vi "graphHandler.vi"(0 "Maxes[wl]":dbl[][](array[numeric]), 4 "Bounds[wl]":dbl[][](array[numeric]), 5 "delta inc":dbl, 6 "deltas":dbl[](array[numeric]), 7 "freq inc":dbl, 8 "wavelengths":dbl[](array[numeric]), 11 "trace (r=wl, c=d)":dbl[][](array[numeric])=array321x127[40767 elements]) -> (1 "Scale mult/offset":T2, 2 "Cursors":T1(array[cluster]), 3 "output trace (r=d, c=freq)":dbl[][](array[numeric]))   [LabVIEW 2022 SP3]
uses:
  <vilib>/gmath/NI_Gmath.lvlib
panel:
  out "resampled deltas":dbl[](array[numeric])
  out "error 2":i32
  out "resampled freqs":dbl[](array[numeric])
  out "Array":dbl[](array[numeric])
  out "error":i32
  out "freqs (rad*PHz)":dbl[](array[numeric])
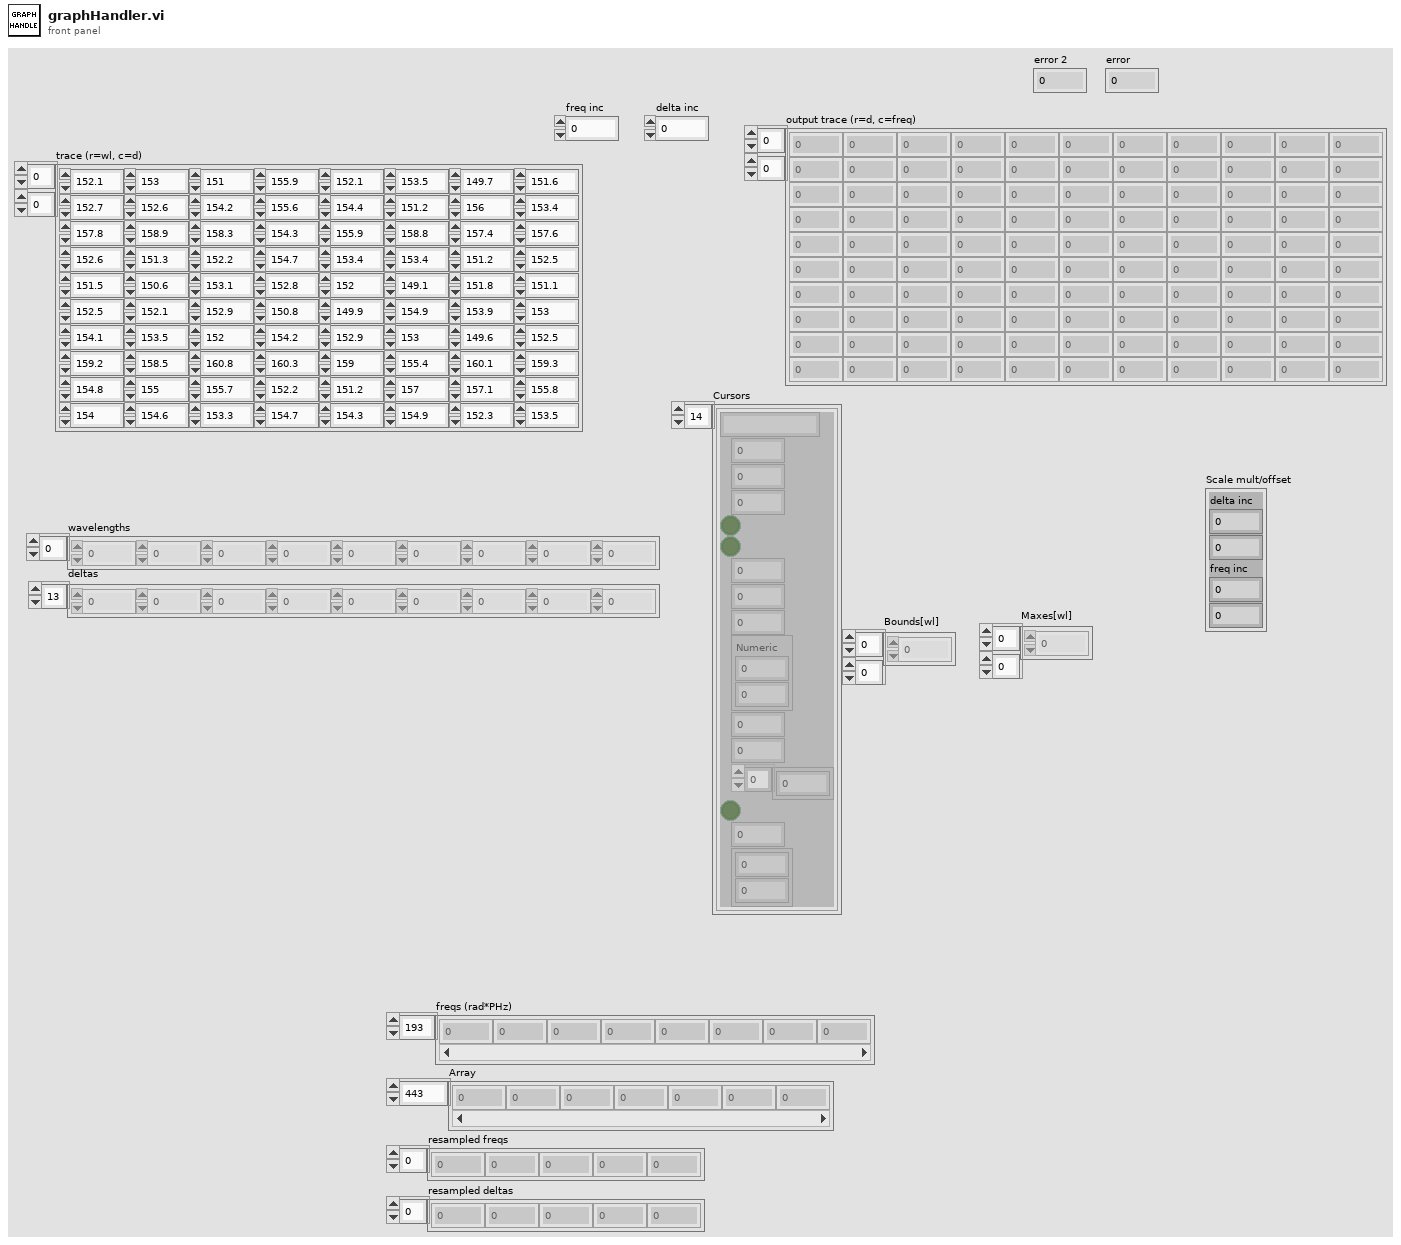
[diagram p1: front panel]
types:
  T1 = cluster{string, i32, i32, i32, bool, bool, i32, i32, i32, cluster{"Numeric":dbl, dbl}, i32, i32, i32[], bool, i32, cluster{dbl, dbl}}[]
  T2 = cluster{"delta inc":dbl, dbl, "freq inc":dbl, dbl}
  T3 = cluster{string, i32, i32, i32, bool, bool, i32, i32, i32, cluster{"Numeric":dbl, dbl}, i32, i32, i32[], bool, i32, cluster{dbl, dbl}}
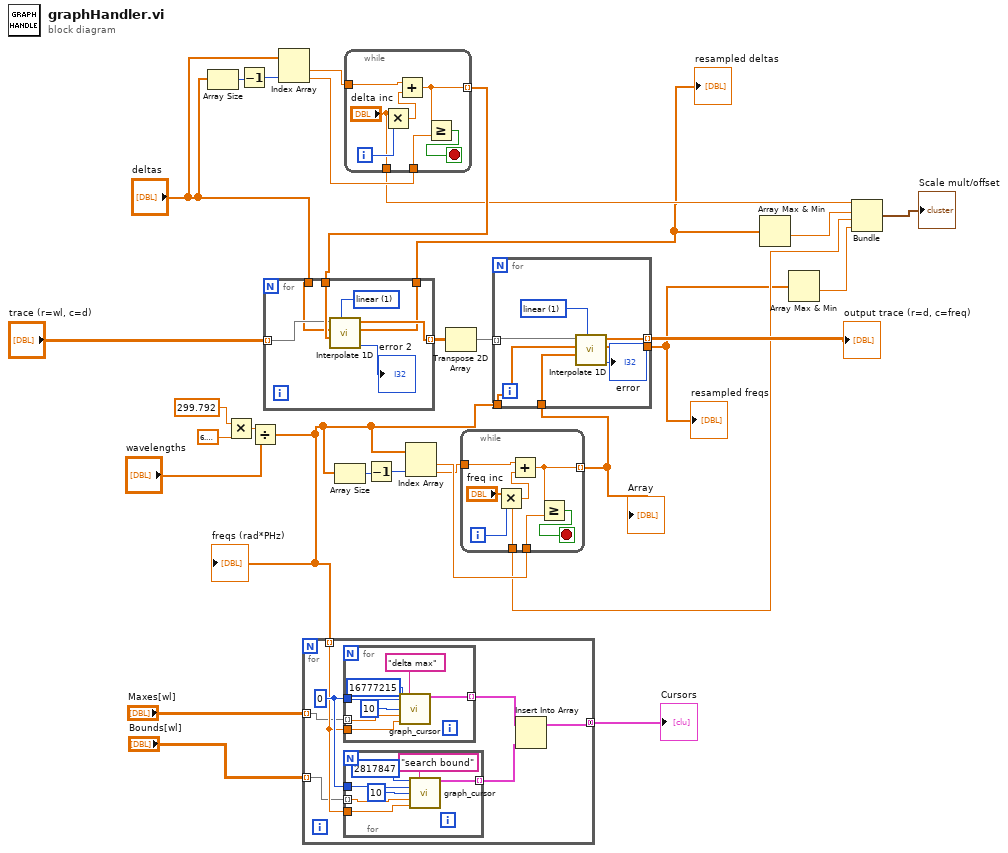
[diagram p0: block diagram]
diagram:
  n1 = Array Size(array="deltas") -> (size(s)=w21:i32)
  n2 = Multiply(x=299.792, y=6.283185307179586) -> (x*y=w28:dbl)
  n3 = Decrement(x=w21) -> (x-1=w20:i32)
  n4 = Divide(x=w28, y="wavelengths") -> (x/y=w6:dbl[])
  "freqs (rad*PHz)" <- w6
  n5 = Index Array(array="deltas", index #2=w20) -> (element #1=w18:dbl, element #2=w19:dbl)  [unwired: 1 in]
  n6 = for {
    tunnel: "Maxes[wl]" -> [w34] mode=indexing
    tunnel: w6 -> [w36] mode=indexing
    tunnel: "Bounds[wl]" -> [w35] mode=indexing
    tunnel: [w31] -> w3 mode=concatenating
    w37 = 0 ("Style")
    n7 = for {
      tunnel: w37 -> [w50]
      tunnel: w36 -> [w45]
      tunnel: w34 -> [w46] mode=indexing
      tunnel: [w47] -> w33 mode=indexing
      n8 = call "graph_cursor.vi"("Colour"=16777215, "Name"="delta max", "Style"=w50, "Point style"=10, "X"=w46, "Y"=w45) -> ("Cursor Cluster"=w47:T3)  [unwired: 9 in]
    }
    n9 = for {
      tunnel: w37 -> [w43]
      tunnel: w36 -> [w38]
      tunnel: w35 -> [w39] mode=indexing
      tunnel: [w40] -> w32 mode=indexing
      n10 = call "graph_cursor.vi"("Colour"=2817847, "Name"="search bound", "Style"=w43, "Point style"=10, "X"=w39, "Y"=w38) -> ("Cursor Cluster"=w40:T3)  [unwired: 9 in]
    }
    n11 = Insert Into Array(array=w33, new element=w32) -> (w31:T1)  [unwired: 1 in]
  }
  "Cursors" <- w3
  n12 = Array Size(array=w6) -> (size(s)=w27:i32)
  n13 = while {
    tunnel: w18 -> [w58]
    tunnel: [w54] -> w16 mode=indexing
    tunnel: w19 -> [w53]
    tunnel: ["delta inc"] -> w13
    i -> [w56]
    stop <- w55 stop-if-true
    n14 = Multiply(x="delta inc", y=w56) -> (x*y=w57:dbl)
    n15 = Add(x=w58, y=w57) -> (x+y=w54:dbl)
    n16 = Greater Or Equal?(x=w54, y=w53) -> (x >= y?=w55:bool)
  }
  n17 = for {
    tunnel: "trace (r=wl, c=d)" -> [w64] mode=indexing
    tunnel: "deltas" -> [w63]
    tunnel: w16 -> [w65]
    tunnel: [w62] -> w15 mode=indexing
    tunnel: [w59] -> w12
    w60 = 1 items=["nearest", "linear", "spline", "cubic Hermite", "Lagrange"] ("method")
    n18 = call <vilib>:"Interpolate 1D.vi"("method"=w60, "xi"=w65, "X"=w63, "Y"=w64) -> ("error"=→"error 2":i32, "xi used"=w59:dbl[], "yi"=w62:dbl[])  [unwired: 5 in]
  }
  "resampled deltas" <- w12
  n19 = Decrement(x=w27) -> (x-1=w26:i32)
  n20 = Index Array(array=w6, index #2=w26) -> (element #1=w23:dbl, element #2=w22:dbl)  [unwired: 1 in]
  n21 = Transpose 2D Array(2D array=w15) -> (transposed array=w24:dbl[][])
  n22 = while {
    tunnel: w22 -> [w72]
    tunnel: [w68] -> w25 mode=indexing
    tunnel: w23 -> [w67]
    tunnel: ["freq inc"] -> w10
    i -> [w70]
    stop <- w69 stop-if-true
    n23 = Multiply(x="freq inc", y=w70) -> (x*y=w71:dbl)
    n24 = Add(x=w72, y=w71) -> (x+y=w68:dbl)
    n25 = Greater Or Equal?(x=w68, y=w67) -> (x >= y?=w69:bool)
  }
  "Array" <- w25
  n26 = for {
    tunnel: w24 -> [w79] mode=indexing
    tunnel: w6 -> [w78]
    tunnel: w25 -> [w77]
    tunnel: [w75] -> w14 mode=indexing
    tunnel: [w74] -> w9
    w76 = 1 items=["nearest", "linear", "spline", "cubic Hermite", "Lagrange"] ("method")
    n27 = call <vilib>:"Interpolate 1D.vi"("method"=w76, "xi"=w77, "X"=w78, "Y"=w79) -> ("error"=→"error":i32, "xi used"=w74:dbl[], "yi"=w75:dbl[])  [unwired: 5 in]
  }
  "output trace (r=d, c=freq)" <- w14
  "resampled freqs" <- w9
  n28 = Array Max & Min(array=w12) -> (min value=w11:dbl)  [unwired: 3 out]
  n29 = Array Max & Min(array=w9) -> (min value=w8:dbl)  [unwired: 3 out]
  n30 = Bundle("delta inc"=w13, w11, "freq inc"=w10, w8) -> (→"Scale mult/offset":T2)  [unwired: 1 in]
